vi "Read Terminals.vi"(6 "parameters file version":string, 8 "error in":errorcluster, 11 "channel ref in":refnum<k20>) -> (0 "error out":errorcluster, 1 "terminal names":string[](array[string]), 2 "terminal addresses":T1[](array[typedef]), 3 "channel ref out":refnum<k20>)   [LabVIEW 2020, in "MIL-STD 1553 Import.lvlib"]
uses:
  MIL-STD 1553 Import.lvlib
  Shared/Address.ctl
  67bcb88d-b419-4137-882e-0df92e3c6eb4.vi
  75fac746-238b-4eff-9e8c-95883f48f3c9.vi
  67bcb88d-b419-4137-882e-0df92e3c6eb4.vi/b1e6fcf8-dac1-42d2-b1fe-151afe06dbd4.vi
  75fac746-238b-4eff-9e8c-95883f48f3c9.vi/b1e6fcf8-dac1-42d2-b1fe-151afe06dbd4.vi
  67bcb88d-b419-4137-882e-0df92e3c6eb4.vi/b1e6fcf8-dac1-42d2-b1fe-151afe06dbd4.vi/49c1b1ee-2d2a-4a85-8ca5-42123c34e85a.vi
  Constants.vi
  <vilib>/xml/Get Node Text Content.vi
  <vilib>/Utility/error.llb/Error Cluster From Error Code.vi
  Scripting/Constants.vi
  Scripting/Ballard MIL-STD-1553 Scripting.lvlib
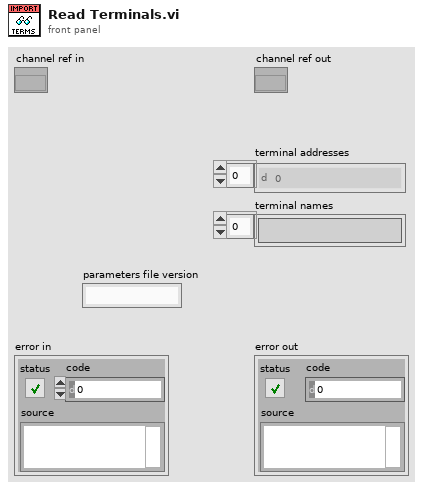
[diagram p1: front panel]
types:
  T1 = typedef "Address.ctl" = u16
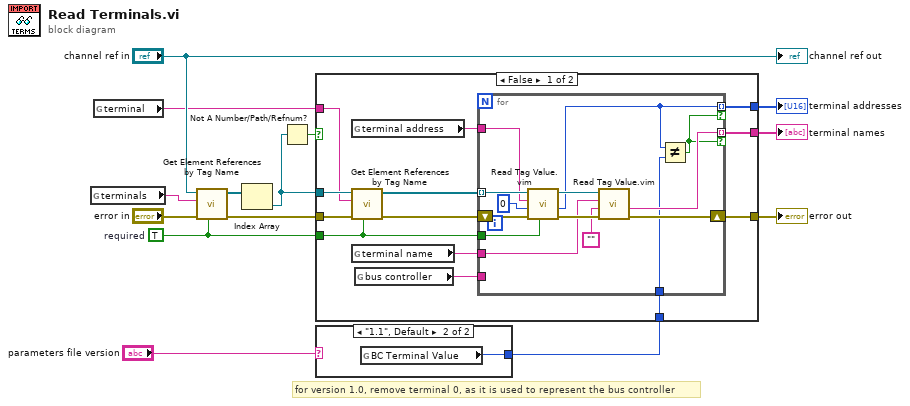
[diagram p0: block diagram]
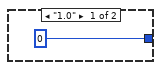
[diagram p2: hidden frame]
diagram:
  w6 = TRUE  # required
  # "for version 1.0, remove terminal 0, as it is used to represent the bus controller"
  n1 = global read "Constants.vi" "terminals"() -> (w5:string)
  n2 = global read "Constants.vi" "terminal"() -> (w4:string)
  n3 = call "Get Element References by Tag Name.vi"("required (F)"=w6, "error in"="error in", "tag name"=w5, "node in"="channel ref in") -> ("error out"=w9:errorcluster, "array of elements"=w10:refnum<k20>[])  [unwired: 6 in]
  n4 = Index Array(array=w10) -> (element=w7:refnum<k20>)  [unwired: 1 in]
  n5 = Not A Number/Path/Refnum?(number/path/refnum=w7) -> (NaN/Path/Refnum?=w8:bool)
  n6 = case shown="\"1.1\", Default" "parameters file version" {
    tunnel: [0 w16] -> w1
    frame "1.0" {
    }
    frame "1.1", Default {
      n7 = global read "Constants.vi" "BC Terminal Value"() -> (w16:u16)
    }
  }
  n8 = case shown="False" w8 {
    tunnel: [w29 w44] -> w14
    tunnel: [w28 _] -> w11
    tunnel: w7 -> [w27 _]
    tunnel: w9 -> [w26 w44]
    tunnel: w6 -> [w21 _]
    tunnel: w4 -> [w25 _]
    tunnel: [w19 _] -> w3
    tunnel: w1 -> [w17 _]
    frame False {
      n9 = global read "Constants.vi" "terminal address"() -> (w22:string)
      n10 = call "Get Element References by Tag Name.vi"("required (F)"=w21, "error in"=w26, "tag name"=w25, "node in"=w27) -> ("error out"=w23:errorcluster, "array of elements"=w24:refnum<k20>[])  [unwired: 6 in]
      n11 = global read "Constants.vi" "terminal name"() -> (w20:string)
      n12 = global read "Constants.vi" "bus controller"() -> (w18:string)
      n13 = for {
        shift-right: [w33] -> w29
        shift-left: w23 -> [w42]
        tunnel: [w31] -> w28 mode=indexing if=w30
        tunnel: w24 -> [w43] mode=indexing
        tunnel: w22 -> [w41]
        tunnel: w21 -> [w40]
        tunnel: w20 -> [w36]
        tunnel: [w34] -> w19 mode=indexing if=w30
        tunnel: w18 -> [_]
        tunnel: w17 -> [w32]
        n14 = call "Read Tag Value.vim"("required (F)"=w40, "error in"=w42, "default"=u16 0, "tag name"=w41, "node in"=w43) -> ("error out"=w37:errorcluster, "value"=w31:u16, "node out"=w38:refnum<k20>)  [unwired: 4 in]
        n15 = call "Read Tag Value.vim"("error in"=w37, "default"="", "tag name"=w36, "node in"=w38) -> ("error out"=w33:errorcluster, "value"=w34:string)  [unwired: 5 in, 1 out]
        n16 = Not Equal?(x=w31, y=w32) -> (x != y?=w30:bool)
      }
    }
    frame True {
    }
  }
  "error out" <- w14
  "terminal addresses" <- w11
  "terminal names" <- w3
  "channel ref out" <- "channel ref in"
